vi "CipheredString_to_Cluster.vi"(0 "BitKeyType (256)":u16(ring)=256 items=["AES bit key 128"=128, "AES bit key 192"=192, "AES bit key 256"=256], 1 "password to cipher users":string, 7 "Cyphered text":string, 11 "error in (no error)":errorcluster) -> (4 "String 1":string, 6 "String 2":string, 8 "Time Stamp":timestamp, 10 "Account":T1, 15 "error out":errorcluster)   [LabVIEW 2012]
uses:
  typedef/User Accounts.ctl
panel:
  out "Plain Text":string
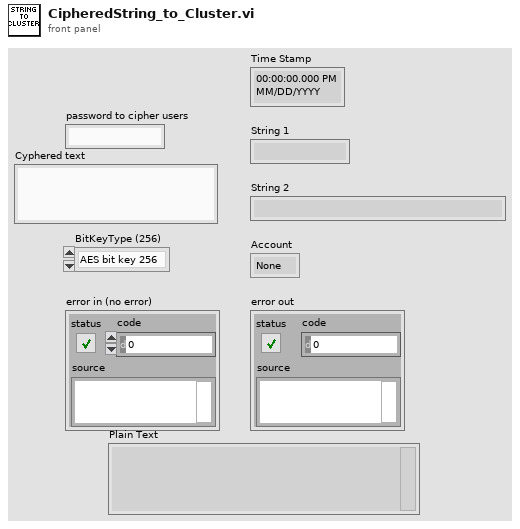
[diagram p1: front panel]
types:
  T1 = typedef "User Accounts.ctl" = enum16{"None", "User", "Admin"}
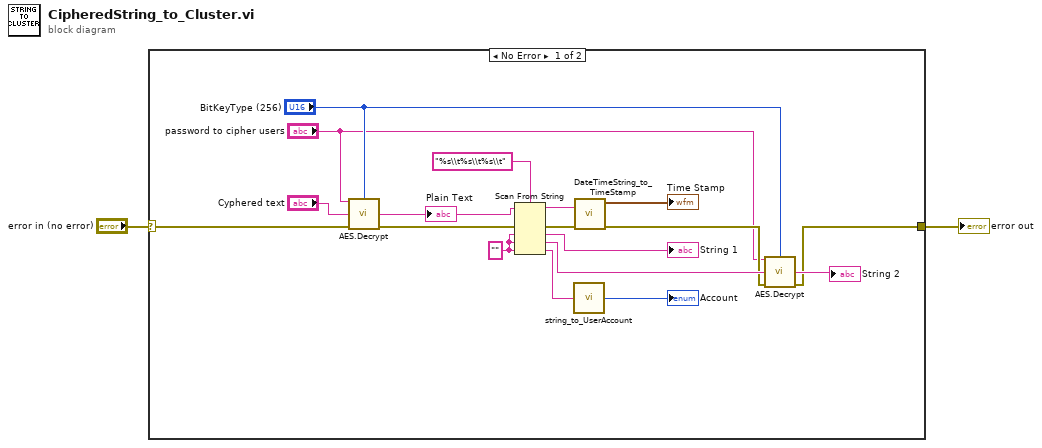
[diagram p0: block diagram]
diagram:
  n1 = case shown="No Error" "error in (no error)" {
    selector: "error in (no error)" -> [w3 w21]
    tunnel: [w6 w21] -> w2
    frame No Error {
      w16 = ""
      n2 = call <vilib>:"AES.Decrypt.vi"("Password"="password to cipher users", "BitKeyType (256)"="BitKeyType (256)", "EncryptedText"="Cyphered text", "error in"=w3) -> ("Plain Text"=w10:string, "error out"=w18:errorcluster)  [unwired: 10 in]
      "Plain Text" <- w10
      n3 = Scan From String(format string="%s\\t%s\\t%s\\t", input string=w10, error in=w18, default 1=w16, default 2=w16, default 3=w16) -> (remaining string=w17:string, error out=w20:errorcluster, output 1=→"String 1":string, output 2=w8:string, output 3=w14:string)  [unwired: 1 in, 1 out]
      n4 = call "string_to_UserAccount.vi"("String account"=w14) -> ("Account"=→"Account":T1)
      n5 = call "DateTimeString_to_TimeStamp.vi"("error in"=w20, "%m/%d/%Y %H:%M:%S string"=w17) -> ("error out"=w7:errorcluster, "Time Stamp"=→"Time Stamp":timestamp)  [unwired: 8 in]
      n6 = call <vilib>:"AES.Decrypt.vi"("Password"="password to cipher users", "BitKeyType (256)"="BitKeyType (256)", "EncryptedText"=w8, "error in"=w7) -> ("Plain Text"=→"String 2":string, "error out"=w6:errorcluster)  [unwired: 10 in]
    }
    frame Error {
    }
  }
  "error out" <- w2
